vi "Get or Add TablePart.vi"(7 "Sheet Name":string, 8 "error in":errorcluster, 10 "TableDefinitionPart in":refnum<k24>, 11 "SpreadsheetDoc in":refnum<k24>) -> (0 "error out":errorcluster, 2 "TablePart":refnum<k24>, 3 "SpreadsheetDo out":refnum<k24>, 5 "Sheet Name":string)   [LabVIEW 2019, in "Open Xml.lvlib"]
uses:
  Open Xml.lvlib
  D:/git/Open-Xml-LabVIEW/Source/DocumentFormat.OpenXml.dll
  DocumentFormat.OpenXml.dll
panel:
  out "TableDefinitionPart out":refnum<k24>
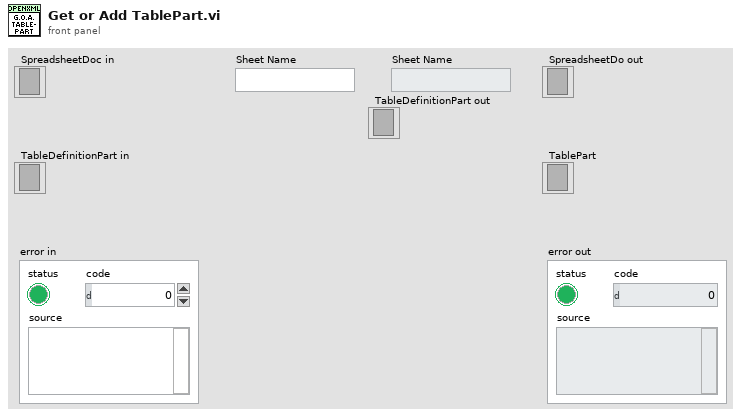
[diagram p1: front panel]
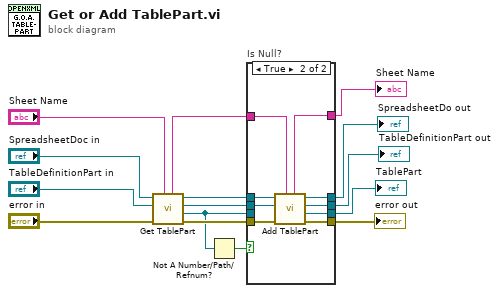
[diagram p0: block diagram]
diagram:
  n1 = call "Get TablePart.vi"("Sheet Name in"="Sheet Name", "error in"="error in", "TableDefinitionPart in"="TableDefinitionPart in", "SpreadsheetDoc in"="SpreadsheetDoc in") -> ("error out"=w13:errorcluster, "TablePart"=w3:refnum<k24>, "TableDefinitionPart out"=w2:refnum<k24>, "SpreadsheetDoc out"=w9:refnum<k24>, "Sheet Name out"=w6:string)  [unwired: 3 in]
  n2 = Not A Number/Path/Refnum?(number/path/refnum=w3) -> (NaN/Path/Refnum?=w10:bool)
  n3 = case "Is Null?" shown="True" w10 {
    tunnel: w13 -> [w18 w29]
    tunnel: [w18 w27] -> w11
    tunnel: w9 -> [w19 w28]
    tunnel: w3 -> [w20 _]
    tunnel: [w20 w22] -> w8
    tunnel: [w19 w26] -> w7
    tunnel: w6 -> [w17 w25]
    tunnel: [w17 w24] -> w5
    tunnel: w2 -> [w16 w23]
    tunnel: [w16 w21] -> w1
    frame False {
    }
    frame True {
      n4 = call "Add TablePart.vi"("Sheet Name"=w25, "error in"=w29, "TableDefinitionPart in"=w23, "SpreadsheetDoc in"=w28) -> ("error out"=w27:errorcluster, "TablePart"=w22:refnum<k24>, "TableDefinitionPart out"=w21:refnum<k24>, "SpreadsheetDoc out"=w26:refnum<k24>, "Sheet Name"=w24:string)  [unwired: 3 in]
    }
  }
  "SpreadsheetDo out" <- w7
  "Sheet Name" <- w5
  "error out" <- w11
  "TablePart" <- w8
  "TableDefinitionPart out" <- w1
